vi "SaveWithZeroGlubina (SubVI).vi"(11 "Table":string[][](array[string])) -> (3 "all rows out":string[][](array[string]))   [LabVIEW 2017]
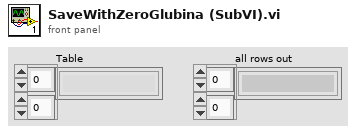
[diagram p1: front panel]
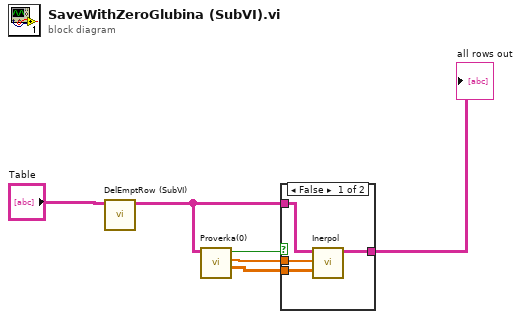
[diagram p0: block diagram]
diagram:
  n1 = call "DelEmptRow (SubVI).vi"("all rows in"="Table") -> ("all rows out"=w2:string[][])  [unwired: 10 in]
  n2 = call "Proverka(0).vi"("all rows"=w2) -> ("ArrayChastot"=w4:dbl[][], "All GLUBIN"=w3:dbl[], "x >= 0?"=w1:bool)  [unwired: 8 in]
  n3 = case shown="False" w1 {
    tunnel: [w7 w11] -> w5
    tunnel: w2 -> [w10 w11]
    tunnel: w3 -> [w9 _]
    tunnel: w4 -> [w8 _]
    frame False {
      n4 = call "Inerpol.vi"("ArrayChastot"=w8, "All GLUBIN"=w9, "all rows"=w10) -> ("appended array"=w7:string[][])  [unwired: 8 in]
    }
    frame True {
    }
  }
  "all rows out" <- w5
